vi "tag select get channel in column.vi"(10 "Column":i32, 11 "tag select name":string) -> (3 "String":string)   [LabVIEW 2013, in "tag select module editor node.lvclass"]
uses:
  tag select module editor node.lvclass
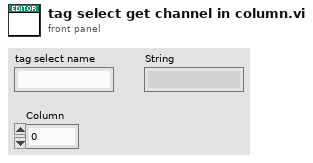
[diagram p1: front panel]
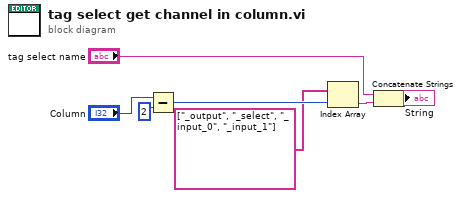
[diagram p0: block diagram]
diagram:
  n1 = Subtract(x="Column", y=2) -> (x-y=w3:i32)
  n2 = Index Array(array=string[] ["_output", "_select", "_input_0", "_input_1"], index=w3) -> (element=w7:string)
  n3 = Concatenate Strings("tag select name", w7) -> (→"String":string)
